vi "Build-timeline.vi"(8 "error in (no error)":errorcluster, 10 "Temp-timeline in":T1, 11 "Set in":refnum<class "Set.lvclass">) -> (0 "error out":errorcluster, 2 "Temp-timeline":T1, 3 "Set out":refnum<class "Set.lvclass">)   [LabVIEW 2013, in "HardwareCharacterization.lvlib" / "Set.lvclass"]
uses:
  Set.lvclass
  ScanParser/Path-buffer.ctl
  ScanParser/Point-buffer.ctl
  Elements.ctl
  ScanParser/Property-buffer.ctl
  ScanParser/Units.ctl
  ScanParser/Speed.ctl
  Element-XML.lvclass/Element-XML.ctl
  Attribute-XML/Attribute-XML.lvclass
  Read Attributes.vi
  Element-XML.lvclass
  ScanParser/HC-ScanParser.lvclass
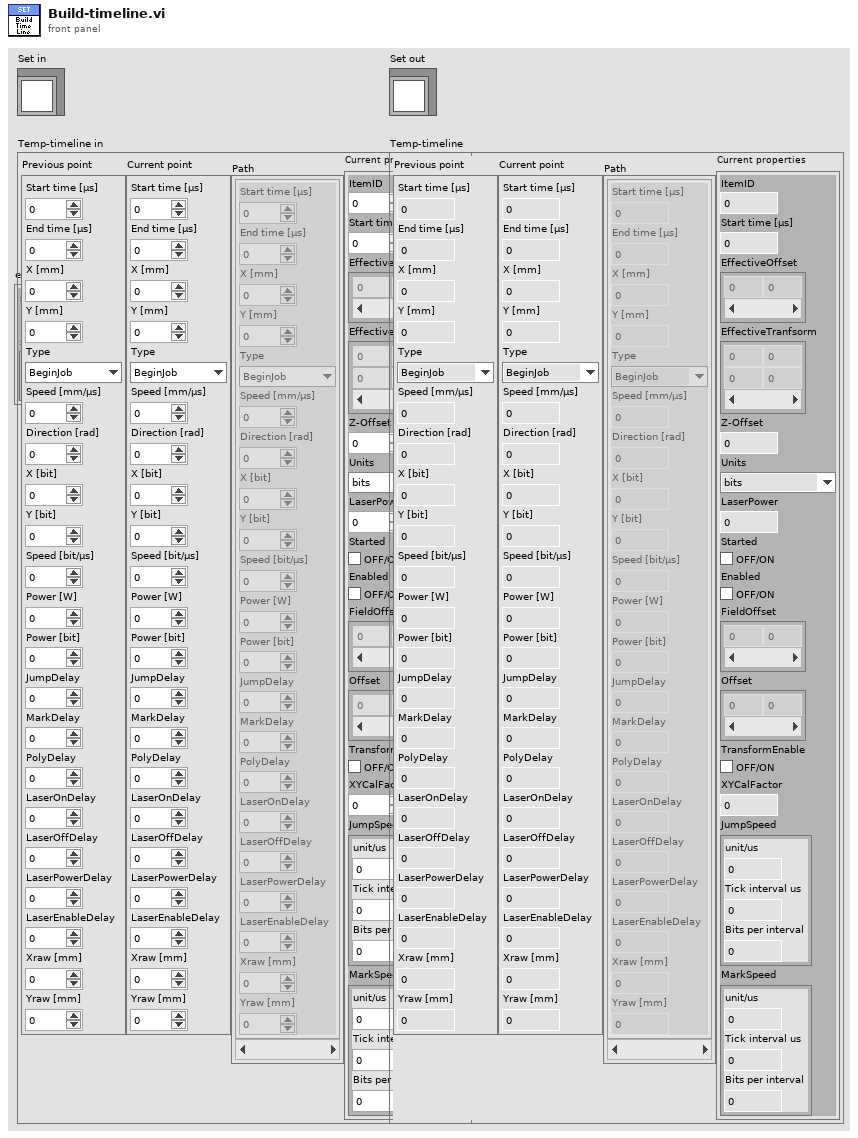
[diagram p1: front panel]
types:
  T1 = typedef "HardwareCharacterization.lvlib/HC-ScanParser.lvclass/Path-buffer.ctl" = cluster{"Previous point":T2, "Current point":T2, "Path":T2[], "Current properties":T4}
  T2 = typedef "HardwareCharacterization.lvlib/HC-ScanParser.lvclass/Point-buffer.ctl" = cluster{"Start time [µs]":i64, "End time [µs]":i64, "X [mm]":dbl, "Y [mm]":dbl, "Type":T3, "Speed [mm/µs]":dbl, "Direction [rad]":dbl, "X [bit]":i16, "Y [bit]":i16, "Speed [bit/µs]":dbl, "Power [W]":dbl, "Power [bit]":u8, "JumpDelay":i64, "MarkDelay":i64, "PolyDelay":i64, "LaserOnDelay":i64, "LaserOffDelay":i64, "LaserPowerDelay":i64, "LaserEnableDelay":i64, "Xraw [mm]":dbl, "Yraw [mm]":dbl}
  T3 = typedef "HardwareCharacterization.lvlib/Element-XML.lvclass/Elements.ctl" = enum16{"BeginJob", "WriteDigital", "WriteAnalog", "Set", "ApplicationEvent", "JumpAbs", "MarkAbs", "JumpRel", "MarkRel", "LongDelay", "EndJob"}
  T4 = typedef "HardwareCharacterization.lvlib/HC-ScanParser.lvclass/Property-buffer.ctl" = cluster{"ItemID":u32, "Start time":i64, "EffectiveOffset":dbl[], "EffectiveTranfsorm":dbl[][], "Z-Offset":sgl, "Units":T5, "LaserPower":u8, "Started":bool, "Enabled":bool, "FieldOffset":dbl[], "Offset":dbl[], "TransformEnable":bool, "XYCalFactor":dbl, "JumpSpeed":T6, "MarkSpeed":T6}
  T5 = typedef "HardwareCharacterization.lvlib/HC-ScanParser.lvclass/Units.ctl" = enum16{"bits", "mm", "inch", "mils"}
  T6 = typedef "HardwareCharacterization.lvlib/HC-ScanParser.lvclass/Speed.ctl" = cluster{"unit/us":dbl, "Tick interval us":u16, "Bits per interval":u16}
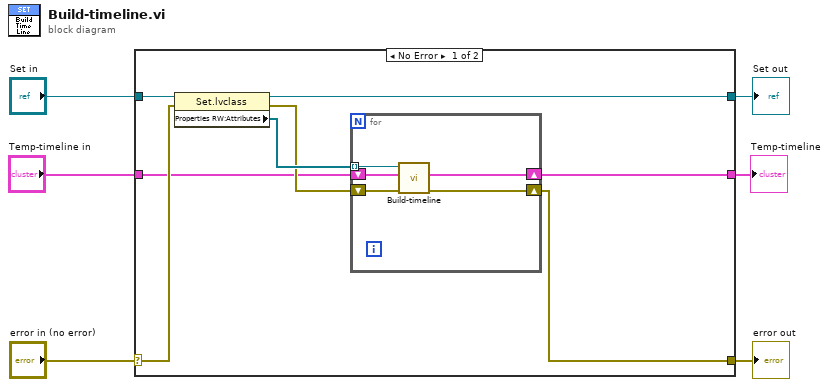
[diagram p0: block diagram]
diagram:
  n1 = case shown="No Error" "error in (no error)" {
    selector: "error in (no error)" -> [w9 w22]
    tunnel: [w8 w22] -> w5
    tunnel: [w13 w21] -> w3
    tunnel: "Set in" -> [w14 w21]
    tunnel: [w10 w20] -> w1
    tunnel: "Temp-timeline in" -> [w7 w20]
    frame No Error {
      n2 = property class="Set.lvclass"(reference=w14, error in=w9) -> (reference out=w13:refnum<class "Set.lvclass">, error out=w11:errorcluster, "Properties RW:Attributes"=w12:refnum<class "Attribute-XML.lvclass">[])
      n3 = for {
        tunnel: w12 -> [w19] mode=indexing
        shift-right: [w15] -> w8
        shift-left: w11 -> [w18]
        shift-right: [w16] -> w10
        shift-left: w7 -> [w17]
        n4 = call-dynamic "Build-timeline.vi"("error in (no error)"=w18, "Temp-timeline in"=w17, "Attribute in"=w19) -> ("error out"=w15:errorcluster, "Temp-timeline"=w16:T1)  [unwired: 6 in, 1 out]
      }
    }
    frame Error {
    }
  }
  "error out" <- w5
  "Set out" <- w3
  "Temp-timeline" <- w1
